vi "Test Read.vi"() -> ()   [LabVIEW 2020]
uses:
  GPS/GPS.lvclass
  C:/Users/dzoni/Documents/NJ/Playground/LV/TCP GPS/lv_tcp_gps/TCP/TCP.lvclass
  TCP/TCP.lvclass/TCP.ctl
  4bec4c2f-f971-4ce2-8ee6-93cbad333557.vi
  TCP/TCP.lvclass
panel:
  in  "Stop":bool
  out "ID":string
  out "Port":u16
  out "Data":string
  out "Address":string
  out "error out":errorcluster
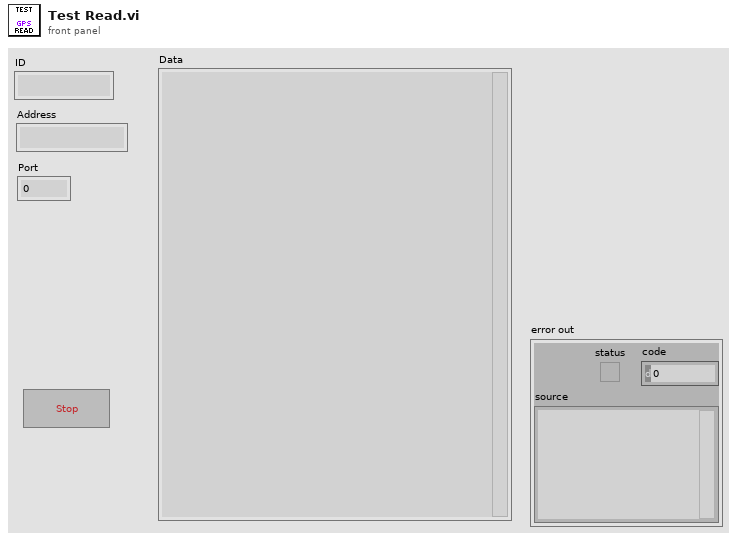
[diagram p1: front panel]
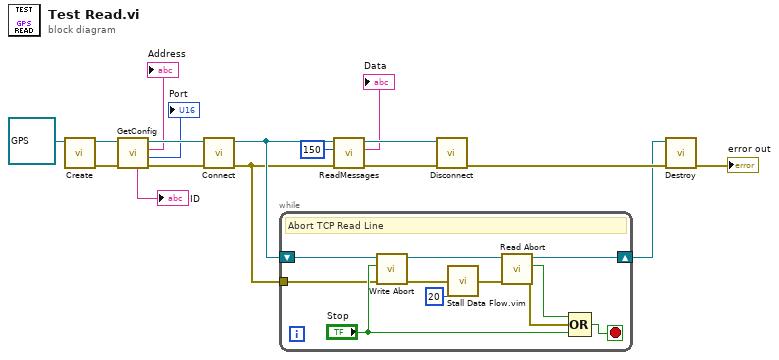
[diagram p0: block diagram]
diagram:
  n1 = call-dynamic "Create.vi"("GPS in"=refnum<class "GPS.lvclass"> refnum ("ClientApp1 in")) -> ("error out"=w11:errorcluster, "GPS out"=w13:refnum<class "GPS.lvclass">)  [unwired: 9 in]
  n2 = call "GetConfig.vi"("error in (no error)"=w11, "ClientBase in"=w13) -> ("error out"=w10:errorcluster, "Port"=→"Port":u16, "Address"=→"Address":string, "ClientBase out"=w12:refnum<class "GPS.lvclass">, "ID"=→"ID":string)  [unwired: 5 in]
  n3 = call "Connect.vi"("error in (no error)"=w10, "ClientBase in"=w12) -> ("error out"=w2:errorcluster, "ClientBase out"=w3:refnum<class "GPS.lvclass">)  [unwired: 8 in]
  n4 = while {
    shift-right: [w25] -> w1
    shift-left: w3 -> [w28]
    tunnel: w2 -> [w23]
    stop <- w24 stop-if-true
    # "Abort TCP Read Line"
    n5 = call "Write Abort.vi"("error in (no error)"=w23, "Abort"="Stop", "ClientBase in"=w28) -> ("error out"=w21:errorcluster, "ClientBase out"=w26:refnum<class "GPS.lvclass">)  [unwired: 7 in]
    n6 = call "Stall Data Flow.vim"("value in"=w21, "milliseconds to wait"=u32 20) -> ("value out"=w20:errorcluster)  [unwired: 1 out]
    n7 = call "Read Abort.vi"("error in (no error)"=w20, "ClientBase in"=w26) -> ("error out"=w18:errorcluster, "Abort"=w19:bool, "ClientBase out"=w25:refnum<class "GPS.lvclass">)  [unwired: 7 in]
    n8 = Compound Arithmetic op=OR(w19, w18, "Stop") -> (w24:bool)
  }
  n9 = call "ReadMessages.vi"("error in (no error)"=w2, "NumOfMessages"=150, "GPS in"=w3) -> ("error out"=w16:errorcluster, "Data"=→"Data":string, "GPS out"=w17:refnum<class "GPS.lvclass">)  [unwired: 6 in]
  n10 = call-dynamic "Disconnect.vi"("error in (no error)"=w16, "ClientBase in"=w17) -> ("error out"=w15:errorcluster)  [unwired: 8 in, 1 out]
  n11 = call-dynamic "Destroy.vi"("error in (no error)"=w15, "ClientBase in"=w1) -> ("error out"=→"error out":errorcluster)  [unwired: 9 in]
